vi "Autonomous Independent.vi"   [LabVIEW 2011]
doc: "This VI is called when autonomous begins, and will automatically be terminated when autonomous ends. You can carry out timed or sensor driven robot movement independently without needing to return to the caller."
uses:
  <vilib>/Rock Robotics/WPI/Solenoid/WPI_SolenoidValue.ctl
  Robot Global Data.vi
  <vilib>/Rock Robotics/WPI/Solenoid/WPI_SolenoidSetEnum.vi
  <vilib>/Rock Robotics/WPI/RobotDrive/WPI_RobotDriveArcadeDrive_Standard(NoSaturation).vi
types:
  T1 = typedef "WPI_MotorControlDeviceRef.ctl" = cluster{"DeviceStatus":errorcluster, "Type":enum16{"PWM", "CAN"}, "PWM":cluster{"Digital Module":T2, "PWM Channel":T3, "DeadBand":T4}, "CAN":cluster{"Device Number":u8, "Control Mode":T5, "Semaphore":T6, "Max Vout":dbl}, "Invert":bool, "TransformRef":T7, "InvTransformRef":T7}
  T2 = typedef "FPGA_TypedefDigitalModule.ctl" = enum16{"Digital Module 1", "Digital Module 2"}
  T3 = typedef "FPGA_DIOPWMChannel.ctl" = enum8{"PWM 1", "PWM 2", "PWM 3", "PWM 4", "PWM 5", "PWM 6", "PWM 7", "PWM 8", "PWM 9", "PWM 10", "Invalid"}
  T4 = typedef "WPI_PWMDeadband.ctl" = cluster{"Name":string, "maxPositivePwm":i32, "minPositivePwm":i32, "centerPwm":i32, "maxNegativePwm":i32, "minNegativePwm":i32, "angularRange":u16}
  T5 = typedef "WPI_CANJaguar_ControlMode.ctl" = enum8{"Percent VBus", "Current", "Speed", "Position", "Voltage"}
  T6 = typedef "Semaphore RefNum" = refnum<k1>
  T7 = typedef "WPI_PWMTransform_ConPane.ctl" = refnum<vi>
  T8 = typedef "WPI_RobotDriveDevRef.ctl" = cluster{"DevStatus":errorcluster, "Motors[]":T1[], "Square Inputs":bool, "Max Output":dbl, "Isochronous":bool}
  T9 = typedef "WPI_SolenoidValue.ctl" = enum16{"Off", "On", "Forward", "Reverse"}
  T10 = typedef "WPI_SolenoidDevRef.ctl" = cluster{"DevStatus":errorcluster, "Solenoid Module":T11, "Forward Solenoid Channel":T12, "Reverse Solenoid Channel":T12}
  T11 = typedef "FPGA_TypedefSolenoidModule.ctl" = enum16{"Solenoid Module 1", "Solenoid Module 2"}
  T12 = typedef "WPI_SolenoidChannel.ctl" = enum8{"Solenoid 1", "Solenoid 2", "Solenoid 3", "Solenoid 4", "Solenoid 5", "Solenoid 6", "Solenoid 7", "Solenoid 8", "Invalid"}
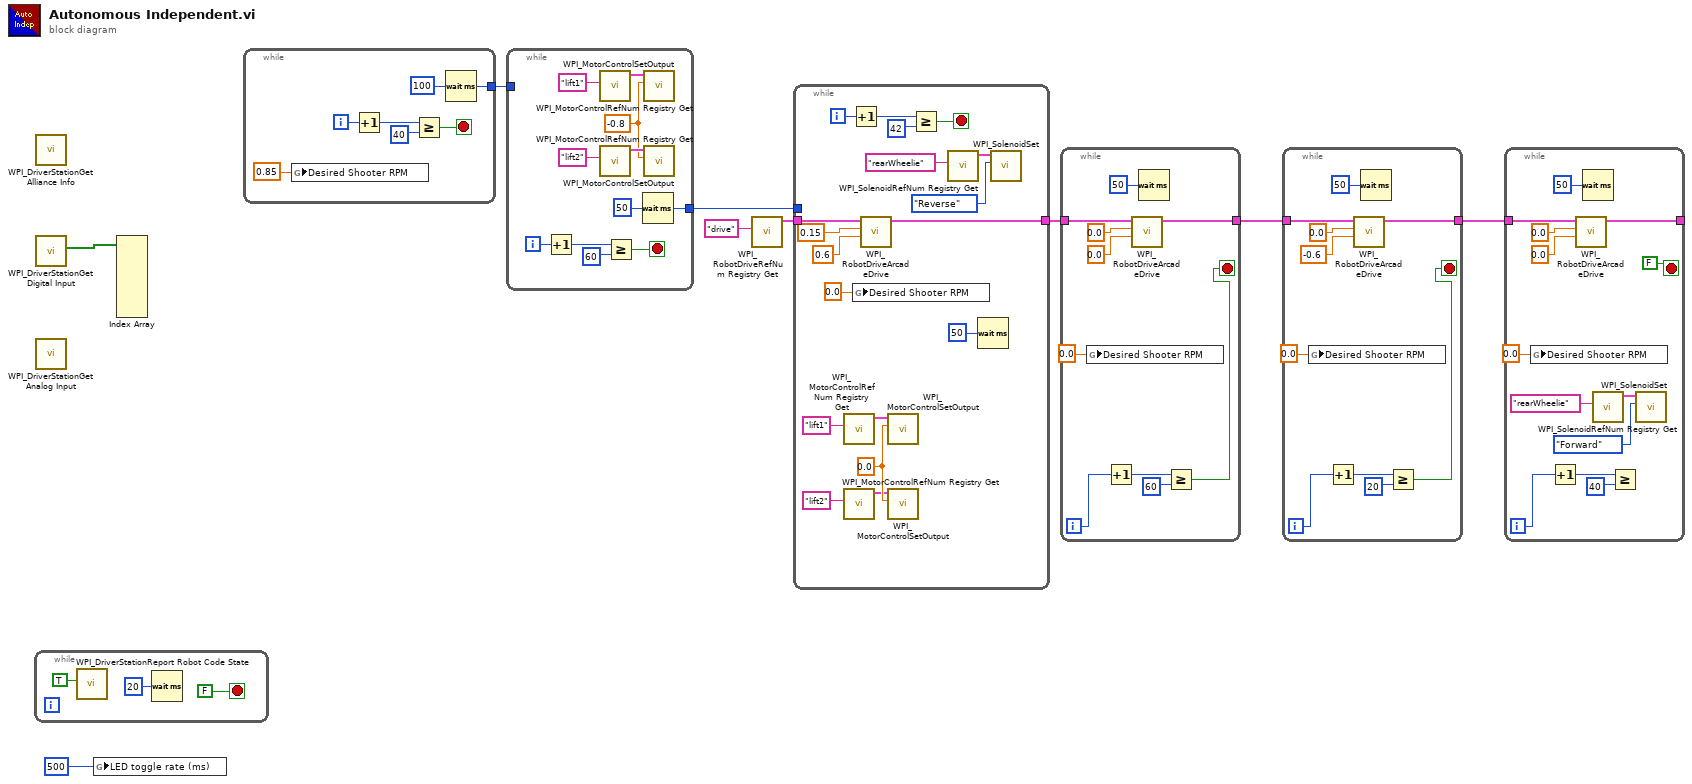
[diagram p0: block diagram]
diagram:
  n1 = while {
    stop <- FALSE stop-if-true
    n2 = call <vilib>:"WPI_DriverStationReport Robot Code State.vi"("Autonomous"=TRUE) -> ()  [unwired: 10 in, 1 out]
    n3 = Wait (ms)(milliseconds to wait=u32 20) -> ()  [unwired: 1 out]
  }
  n4 = call <vilib>:"WPI_DriverStationGet Alliance Info.vi"() -> ()  [unwired: 12 out]
  n5 = call <vilib>:"WPI_DriverStationGet Digital Input.vi"() -> ("Driver Station Digital Input (1-8)"=w9:bool[])  [unwired: 11 out]
  n6 = call <vilib>:"WPI_DriverStationGet Analog Input.vi"() -> ()  [unwired: 12 out]
  n7 = global write "Robot Global Data.vi" "LED toggle rate (ms)"(u32 500 ("LED ms toggle rate")) -> ()
  n8 = Index Array(array=w9) -> ()  [unwired: 8 in, 8 out]
  n9 = while {
    tunnel: [w13] -> w4
    i -> [w16]
    stop <- w14 stop-if-true
    n10 = global write "Robot Global Data.vi" "Desired Shooter RPM"(0.85 ("Desired Shooter RPM")) -> ()
    n11 = Increment(x=w16) -> (x+1=w18:i32)
    n12 = Greater Or Equal?(x=w18, y=40) -> (x >= y?=w14:bool)
    n13 = Wait (ms)(milliseconds to wait=u32 100) -> (millisecond timer value=w13:u32)
  }
  n14 = while {
    tunnel: [w25] -> w3
    tunnel: w4 -> [_]
    i -> [w28]
    stop <- w26 stop-if-true
    w20 = -0.8 ("Output")
    n15 = Increment(x=w28) -> (x+1=w30:i32)
    n16 = call <vilib>:"WPI_MotorControlRefNum Registry Get.vi"("refnum name"="lift1") -> ("MotorControlDevRef"=w21:T1)  [unwired: 9 in, 1 out]
    n17 = call <vilib>:"WPI_MotorControlRefNum Registry Get.vi"("refnum name"="lift2") -> ("MotorControlDevRef"=w22:T1)  [unwired: 9 in, 1 out]
    n18 = Greater Or Equal?(x=w30, y=60) -> (x >= y?=w26:bool)
    n19 = Wait (ms)(milliseconds to wait=u32 50) -> (millisecond timer value=w25:u32)
    n20 = call <vilib>:"WPI_MotorControlSetOutput.vi"("Output"=w20, "MotorControlDevRef"=w21) -> ()  [unwired: 8 in, 2 out]
    n21 = call <vilib>:"WPI_MotorControlSetOutput.vi"("Output"=w20, "MotorControlDevRef"=w22) -> ()  [unwired: 8 in, 2 out]
  }
  n22 = call <vilib>:"WPI_RobotDriveRefNum Registry Get.vi"("refnum name"="drive") -> ("RobotDriveDevRef"=w6:T8)  [unwired: 1 in, 9 out]
  n23 = while {
    tunnel: w6 -> [w48]
    tunnel: [w42] -> w5
    tunnel: w3 -> [_]
    i -> [w45]
    stop <- w43 stop-if-true
    w35 = 0.0 ("Output")
    n24 = call <vilib>:"WPI_MotorControlRefNum Registry Get.vi"("refnum name"="lift1") -> ("MotorControlDevRef"=w34:T1)  [unwired: 9 in, 1 out]
    n25 = call <vilib>:"WPI_MotorControlRefNum Registry Get.vi"("refnum name"="lift2") -> ("MotorControlDevRef"=w33:T1)  [unwired: 9 in, 1 out]
    n26 = Increment(x=w45) -> (x+1=w41:i32)
    n27 = global write "Robot Global Data.vi" "Desired Shooter RPM"(0.0 ("Desired Shooter RPM")) -> ()
    n28 = call-poly <vilib>:"WPI_RobotDriveArcadeDrive.vi"("Y axis value"=0.6 ("X axis value"), "X axis value"=0.15, "RobotDriveDevRef"=w48) -> ("RobotDriveDevRef"=w42:T8)  [unwired: 1 in, 7 out]
    n29 = call <vilib>:"WPI_MotorControlSetOutput.vi"("Output"=w35, "MotorControlDevRef"=w34) -> ()  [unwired: 8 in, 2 out]
    n30 = call <vilib>:"WPI_MotorControlSetOutput.vi"("Output"=w35, "MotorControlDevRef"=w33) -> ()  [unwired: 8 in, 2 out]
    n31 = Greater Or Equal?(x=w41, y=42) -> (x >= y?=w43:bool)
    n32 = call <vilib>:"WPI_SolenoidRefNum Registry Get.vi"("refnum name"="rearWheelie") -> ("SolenoidDevRef"=w39:T10)  [unwired: 9 in, 1 out]
    n33 = Wait (ms)(milliseconds to wait=u32 50) -> ()  [unwired: 1 out]
    n34 = call-poly <vilib>:"WPI_SolenoidSet.vi"("Value"=WPI_SolenoidValue."Reverse", "SolenoidDevRef"=w39) -> ()  [unwired: 8 in, 2 out]
  }
  n35 = while {
    tunnel: w5 -> [w58]
    tunnel: [w54] -> w2
    i -> [w50]
    stop <- w49 stop-if-true
    n36 = global write "Robot Global Data.vi" "Desired Shooter RPM"(0.0 ("Desired Shooter RPM")) -> ()
    n37 = Increment(x=w50) -> (x+1=w52:i32)
    n38 = call-poly <vilib>:"WPI_RobotDriveArcadeDrive.vi"("Y axis value"=0.0 ("X axis value"), "X axis value"=0.0, "RobotDriveDevRef"=w58) -> ("RobotDriveDevRef"=w54:T8)  [unwired: 1 in, 7 out]
    n39 = Wait (ms)(milliseconds to wait=u32 50) -> ()  [unwired: 1 out]
    n40 = Greater Or Equal?(x=w52, y=60) -> (x >= y?=w49:bool)
  }
  n41 = while {
    tunnel: w2 -> [w68]
    tunnel: [w64] -> w1
    i -> [w60]
    stop <- w59 stop-if-true
    n42 = global write "Robot Global Data.vi" "Desired Shooter RPM"(0.0 ("Desired Shooter RPM")) -> ()
    n43 = Increment(x=w60) -> (x+1=w62:i32)
    n44 = call-poly <vilib>:"WPI_RobotDriveArcadeDrive.vi"("Y axis value"=-0.6 ("X axis value"), "X axis value"=0.0, "RobotDriveDevRef"=w68) -> ("RobotDriveDevRef"=w64:T8)  [unwired: 1 in, 7 out]
    n45 = Wait (ms)(milliseconds to wait=u32 50) -> ()  [unwired: 1 out]
    n46 = Greater Or Equal?(x=w62, y=20) -> (x >= y?=w59:bool)
  }
  n47 = while {
    tunnel: w1 -> [w81]
    tunnel: [w77] -> _
    i -> [w72]
    stop <- FALSE stop-if-true
    n48 = global write "Robot Global Data.vi" "Desired Shooter RPM"(0.0 ("Desired Shooter RPM")) -> ()
    n49 = Increment(x=w72) -> (x+1=w74:i32)
    n50 = call-poly <vilib>:"WPI_RobotDriveArcadeDrive.vi"("Y axis value"=0.0 ("X axis value"), "X axis value"=0.0, "RobotDriveDevRef"=w81) -> ("RobotDriveDevRef"=w77:T8)  [unwired: 1 in, 7 out]
    n51 = Wait (ms)(milliseconds to wait=u32 50) -> ()  [unwired: 1 out]
    n52 = call <vilib>:"WPI_SolenoidRefNum Registry Get.vi"("refnum name"="rearWheelie") -> ("SolenoidDevRef"=w71:T10)  [unwired: 9 in, 1 out]
    n53 = Greater Or Equal?(x=w74, y=40) -> ()  [unwired: 1 out]
    n54 = call-poly <vilib>:"WPI_SolenoidSet.vi"("Value"=WPI_SolenoidValue."Forward", "SolenoidDevRef"=w71) -> ()  [unwired: 8 in, 2 out]
  }
